vi "Task Update Message.vi"(8 "error in (no error)":errorcluster, 10 "Task Update Message":string, 11 "BuildServer in":refnum<class "BuildServer.lvclass">) -> (0 "error out":errorcluster, 3 "BuildServer out":refnum<class "BuildServer.lvclass">)   [LabVIEW 2017, in "BuildServer.lvlib" / "BuildServer.lvclass"]
uses:
  BuildServer.lvclass
  BuildServer.lvclass/BuildServer.ctl
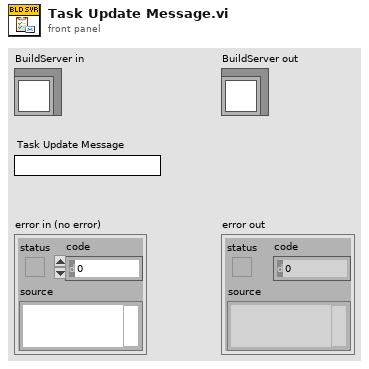
[diagram p1: front panel]
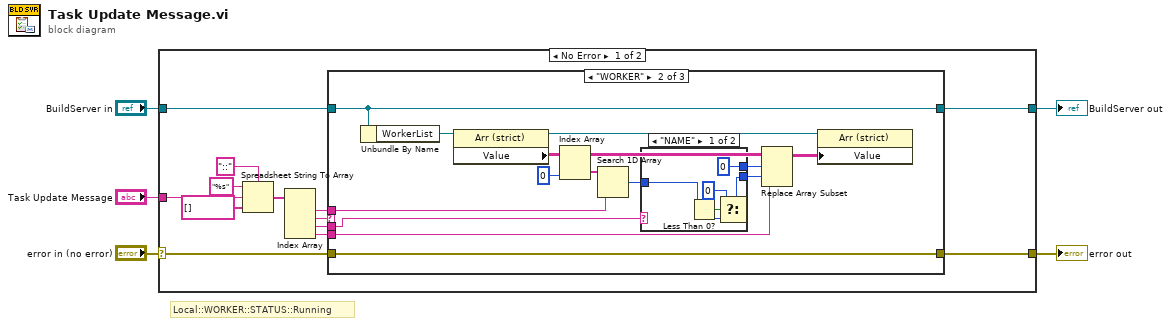
[diagram p0: block diagram]
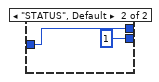
[diagram p3: hidden frame]
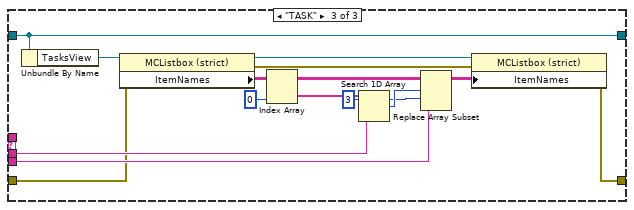
[diagram p4: hidden frame]
diagram:
  # "Local::WORKER::STATUS::Running"
  n1 = case shown="No Error" "error in (no error)" {
    selector: "error in (no error)" -> [w8 w57]
    tunnel: [w7 w57] -> w4
    tunnel: [w9 w56] -> w2
    tunnel: "BuildServer in" -> [w10 w56]
    tunnel: "Task Update Message" -> [w18 _]
    frame No Error {
      n2 = Spreadsheet String To Array(delimiter (Tab)="::", format string="%s", spreadsheet string=w18, array type (2D Dbl)=string[] []) -> (array=w14:string[])
      n3 = Index Array(array=w14) -> (element #1=w6:string, element #2=w13:string, element #3=w12:string, element #4=w11:string)  [unwired: 4 in]
      n4 = case shown="\"WORKER\"" w13 {
        tunnel: w12 -> [_ w23 w52]
        tunnel: w11 -> [_ w27 w48]
        tunnel: w10 -> [w20 w33 w55]
        tunnel: [w20 w33 w55] -> w9
        tunnel: w8 -> [w19 w34 w45]
        tunnel: [w19 w34 w43] -> w7
        tunnel: w6 -> [_ w29 _]
        frame Default {
        }
        frame "WORKER" {
          n5 = Unbundle By Name(w33) -> ("WorkerList"=w32:refnum<vi>)
          n6 = property class="Arr (strict)"(reference=w32) -> (reference out=w26:refnum<vi>, "Value"=w28:string[][])  [unwired: 1 in, 1 out]
          n7 = Index Array(array=w28, index (col)=0 ("disabled index (col)")) -> (element=w30:string[])  [unwired: 1 in]
          n8 = Search 1D Array(1D array=w30, element=w29) -> (index of element=w24:i32)  [unwired: 1 in]
          n9 = case shown="\"NAME\"" w23 {
            tunnel: w24 -> [w38 w40]
            tunnel: [w35 1 ("disabled index (col)")] -> w22
            tunnel: [0 ("disabled index (col)") w40] -> w21
            frame "NAME" {
              n10 = Less Than 0?(x=w38) -> (x < 0?=w39:bool)
              n11 = Select(t=0, s=w39, f=w38) -> (s? t:f=w35:i32)
            }
            frame "STATUS", Default {
            }
          }
          n12 = Replace Array Subset(array=w28, new element=w27, index (row)=w21, index (col)=w22) -> (w25:string[][])
          n13 = property class="Arr (strict)"(reference=w26, "Value"=w25) -> ()  [unwired: 1 in, 2 out]
        }
        frame "TASK" {
          n14 = Unbundle By Name(w55) -> ("TasksView"=w54:refnum<vi>)
          n15 = property class="MCListbox (strict)"(reference=w54, error in=w45) -> (reference out=w47:refnum<vi>, error out=w44:errorcluster, "ItemNames"=w51:string[][])
          n16 = Index Array(array=w51, index (col)=0 ("disabled index (col)")) -> (element=w53:string[])  [unwired: 1 in]
          n17 = Search 1D Array(1D array=w53, element=w52) -> (index of element=w50:i32)  [unwired: 1 in]
          n18 = Replace Array Subset(array=w51, new element=w48, index (row)=w50, index (col)=3 ("disabled index (col)")) -> (w46:string[][])
          n19 = property class="MCListbox (strict)"(reference=w47, error in=w44, "ItemNames"=w46) -> (error out=w43:errorcluster)  [unwired: 1 out]
        }
      }
    }
    frame Error {
    }
  }
  "error out" <- w4
  "BuildServer out" <- w2
